vi "Create Grain.vi"(9 "Grain Size":T1={"Min Length (A)"=10.0, "Max Length (A)"=60.0, "Max Height"=100.0, "Max Width"=100.0, "Grain 1 Start"=0.0, "Tolerance"=0.1}, 10 "Viewing Angle":dbl[](array[numeric])=[1.0, -1.0, 0.0], 11 "Grain Orientation":dbl[](array[numeric])=[1.0, 1.0, 1.0]) -> (3 "Grain":T2={"Structure Name"="CdTe Expanded to Box", "Lattice vector a"=[10.01, 0.0, 0.0], "Lattice vector b"=[0.0, 10.01, 0.0], "Lattice vector c"=[0.0, 0.0, 11.3], "Atoms Array"=[{"Atom Name"="Cd", "Positions (Direct)"=[[0.0, 0.0, 0.0], [0.0, 0.26981849571539923, 0.67603992388645], [0.0, 0.5396369914307985, 0.338019961943225], [0.0, 0.8094554871461977, 0.0], [0.23366967170043837, 0.13490924785769962, 0.338019961943225], [0.23366967170043837, 0.4047277435730989, 0.0], [0.23366967170043837, 0.674546239288498, 0.67603992388645], [0.23366967170043837, 0.9443647350038973, 0.338019961943225], [0.46733934340087674, 0.0, 0.0], [0.46733934340087674, 0.26981849571539923, 0.67603992388645], [0.46733934340087674, 0.5396369914307986, 0.338019961943225], [0.46733934340087674, 0.8094554871461977, 0.0], [0.7010090151013151, 0.13490924785769962, 0.338019961943225], [0.7010090151013151, 0.4047277435730989, 0.0], [0.7010090151013151, 0.674546239288498, 0.67603992388645], [0.7010090151013151, 0.9443647350038973, 0.338019961943225], [0.9346786868017535, 0.0, 0.0], [0.9346786868017535, 0.26981849571539923, 0.67603992388645], [0.9346786868017535, 0.5396369914307985, 0.338019961943225], [0.9346786868017535, 0.8094554871461977, 0.0]], "Positions (Cartesian)"=[[0.0, 0.0, 0.0], [0.0, 2.700883142111146, 7.639251139916884], [0.0, 5.401766284222292, 3.819625569958442], [0.0, 8.10264942633344, 0.0], [2.339033413721388, 1.350441571055573, 3.819625569958442], [2.339033413721388, 4.05132471316672, 0.0], [2.339033413721388, 6.752207855277865, 7.639251139916884], [2.339033413721388, 9.453090997389012, 3.819625569958442], [4.678066827442776, 0.0, 0.0], [4.678066827442776, 2.700883142111146, 7.639251139916884], [4.678066827442776, 5.401766284222293, 3.819625569958442], [4.678066827442776, 8.10264942633344, 0.0], [7.017100241164163, 1.350441571055573, 3.819625569958442], [7.017100241164163, 4.05132471316672, 0.0], [7.017100241164163, 6.752207855277865, 7.639251139916884], [7.017100241164163, 9.453090997389012, 3.819625569958442], [9.356133654885552, 0.0, 0.0], [9.356133654885552, 2.700883142111146, 7.639251139916884], [9.356133654885552, 5.401766284222292, 3.819625569958442], [9.356133654885552, 8.10264942633344, 0.0]]}, {"Atom Name"="Te", "Positions (Direct)"=[[0.0, 0.0, 0.25351497145741875], [0.0, 0.2698184957153993, 0.9295548953438687], [0.0, 0.5396369914307985, 0.5915349334006437], [0.0, 0.8094554871461977, 0.25351497145741886], [0.23366967170043837, 0.1349092478576996, 0.5915349334006438], [0.23366967170043837, 0.40472774357309876, 0.25351497145741886], [0.23366967170043837, 0.674546239288498, 0.9295548953438687], [0.23366967170043837, 0.9443647350038973, 0.5915349334006438], [0.46733934340087674, 4.4364556428577685e-17, 0.25351497145741886], [0.46733934340087674, 0.26981849571539923, 0.9295548953438687], [0.46733934340087674, 0.5396369914307986, 0.5915349334006438], [0.46733934340087674, 0.8094554871461977, 0.25351497145741875], [0.7010090151013151, 0.1349092478576996, 0.5915349334006438], [0.7010090151013151, 0.40472774357309876, 0.25351497145741886], [0.7010090151013151, 0.674546239288498, 0.9295548953438687], [0.7010090151013151, 0.9443647350038973, 0.5915349334006438], [0.9346786868017535, 0.0, 0.25351497145741875], [0.9346786868017535, 0.2698184957153993, 0.9295548953438687], [0.9346786868017535, 0.5396369914307985, 0.5915349334006437], [0.9346786868017535, 0.8094554871461977, 0.25351497145741886]], "Positions (Cartesian)"=[[0.0, 0.0, 2.864719177468832], [0.0, 2.7008831421111466, 10.503970317385717], [0.0, 5.401766284222292, 6.684344747427274], [0.0, 8.10264942633344, 2.864719177468833], [2.339033413721388, 1.3504415710555728, 6.684344747427275], [2.339033413721388, 4.051324713166719, 2.864719177468833], [2.339033413721388, 6.752207855277865, 10.503970317385717], [2.339033413721388, 9.453090997389012, 6.684344747427275], [4.678066827442776, 4.440892098500626e-16, 2.864719177468833], [4.678066827442776, 2.700883142111146, 10.503970317385717], [4.678066827442776, 5.401766284222294, 6.684344747427275], [4.678066827442776, 8.10264942633344, 2.864719177468832], [7.017100241164163, 1.3504415710555728, 6.684344747427275], [7.017100241164163, 4.051324713166719, 2.864719177468833], [7.017100241164163, 6.752207855277865, 10.503970317385717], [7.017100241164163, 9.453090997389012, 6.684344747427275], [9.356133654885552, 0.0, 2.864719177468832], [9.356133654885552, 2.7008831421111466, 10.503970317385717], [9.356133654885552, 5.401766284222292, 6.684344747427274], [9.356133654885552, 8.10264942633344, 2.864719177468833]]}], "# of atoms"=40} {"Atoms Array"."Positions (Cartesian)" format="%#_4f"; "Atoms Array"."Positions (Direct)" format="%#_4f"})   [LabVIEW 2010]
uses:
  <vilib>/Analysis/_algsub.llb/Real Vector Norm.vi
  <vilib>/Analysis/NI_AALPro.lvlib
panel:
  in  "Conventional Unit Cell":T2={"Structure Name"="CdTe", "Lattice vector a"=[6.615785553057252, 0.0, 0.0], "Lattice vector b"=[0.0, 6.615785553057252, 0.0], "Lattice vector c"=[0.0, 0.0, 6.615785553057252], "Atoms Array"=[{"Atom Name"="Cd", "Positions (Direct)"=[[0.0, 0.0, 0.0], [0.0, 0.5, 0.5], [0.5, 0.0, 0.5], [0.5, 0.5, 0.0]], "Positions (Cartesian)"=[[0.0, 0.0, 0.0], [0.0, 3.307892776528626, 3.307892776528626], [3.307892776528626, 0.0, 3.307892776528626], [3.307892776528626, 3.307892776528626, 0.0]]}, {"Atom Name"="Te", "Positions (Direct)"=[[0.25, 0.25, 0.25], [0.75, 0.75, 0.25], [0.75, 0.25, 0.75], [0.25, 0.75, 0.75]], "Positions (Cartesian)"=[[1.653946388264313, 1.653946388264313, 1.653946388264313], [4.96183916479294, 4.96183916479294, 1.653946388264313], [4.96183916479294, 1.653946388264313, 4.96183916479294], [1.653946388264313, 4.96183916479294, 4.96183916479294]]}], "# of atoms"=8}
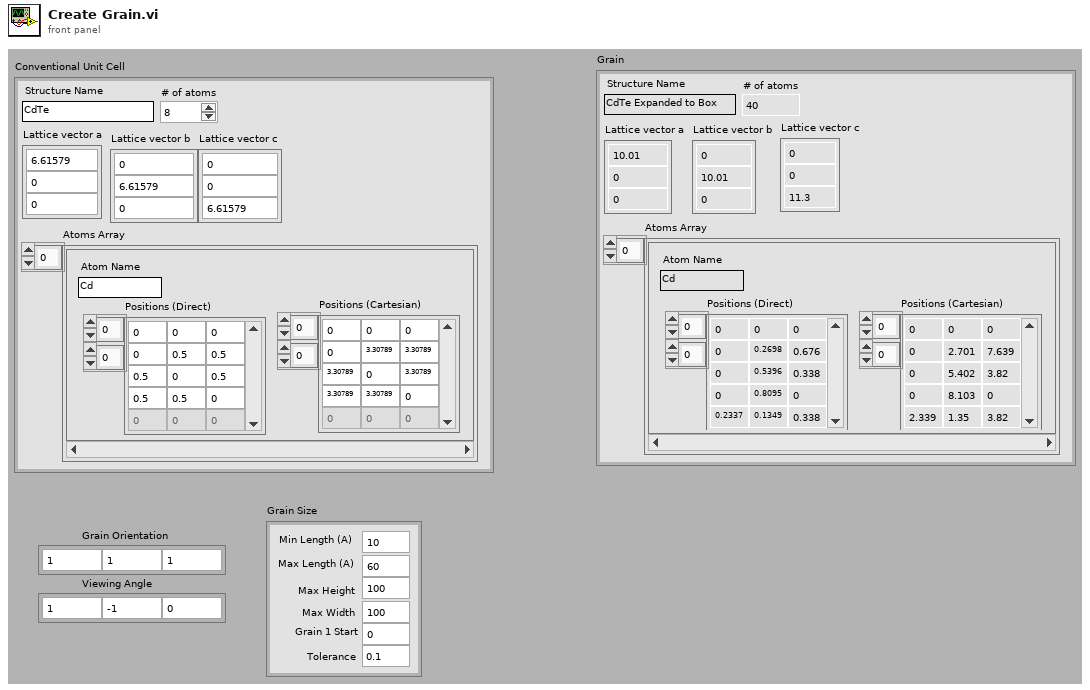
[diagram p1: front panel]
types:
  T1 = cluster{"Min Length (A)":dbl, "Max Length (A)":dbl, "Max Height":dbl, "Max Width":dbl, "Grain 1 Start":dbl, "Tolerance":dbl}
  T2 = cluster{"Structure Name":string, "Lattice vector a":dbl[], "Lattice vector b":dbl[], "Lattice vector c":dbl[], "Atoms Array":cluster{"Atom Name":string, "Positions (Direct)":dbl[][], "Positions (Cartesian)":dbl[][]}[], "# of atoms":i32}
  T3 = typedef "NI_Matrix.lvlib/RealMatrix.ctl" = dbl[][]
  T4 = cluster{dbl, "Max Width":dbl, dbl, "Max Height":dbl, "Grain 1 Start":dbl, "Max Length (A)":dbl}
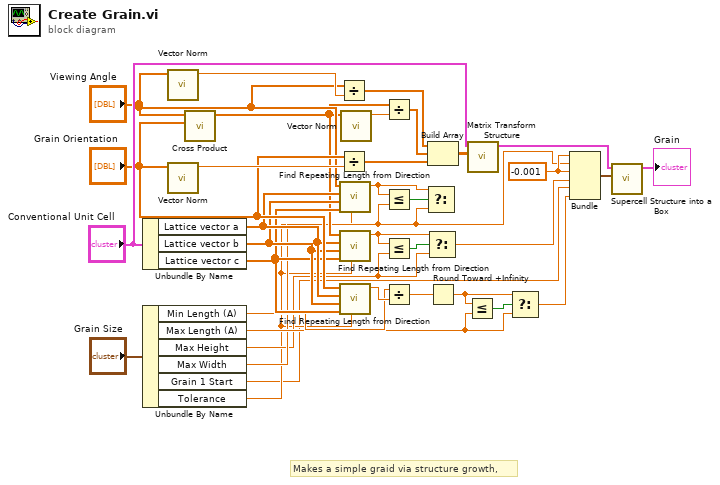
[diagram p0: block diagram]
diagram:
  w10 = -0.001
  # "Makes a simple graid via structure growth,"
  n1 = Unbundle By Name("Conventional Unit Cell") -> ("Lattice vector a"=w21:dbl[], "Lattice vector b"=w20:dbl[], "Lattice vector c"=w19:dbl[])
  n2 = Unbundle By Name("Grain Size") -> ("Min Length (A)"=w6:dbl, "Max Length (A)"=w5:dbl, "Max Height"=w3:dbl, "Max Width"=w4:dbl, "Grain 1 Start"=w1:dbl, "Tolerance"=w2:dbl)
  n3 = call-poly <vilib>:"Vector Norm.vi"("Input Vector"="Viewing Angle") -> ("norm"=w35:dbl)  [unwired: 9 in, 1 out]
  n4 = call-poly <vilib>:"Vector Norm.vi"("Input Vector"="Grain Orientation") -> ("norm"=w33:dbl)  [unwired: 9 in, 1 out]
  n5 = call <vilib>:"Cross Product.vi"("B Vector"="Grain Orientation", "A Vector"="Viewing Angle") -> ("Cross Product"=w17:dbl[])  [unwired: 8 in, 1 out]
  n6 = Divide(x="Viewing Angle", y=w35) -> (x/y=w32:dbl[])
  n7 = Divide(x="Grain Orientation", y=w33) -> (x/y=w31:dbl[])
  n8 = call "Find Repeating Length from Direction.vi"("Tolerance"=w2, "Lattice vector c"=w19, "Lattice vector b"=w20, "Lattice vector a"=w21, "Direction"="Viewing Angle") -> ("Repeating Length (A)"=w15:dbl)  [unwired: 6 in]
  n9 = call "Find Repeating Length from Direction.vi"("Tolerance"=w2, "Lattice vector c"=w19, "Lattice vector b"=w20, "Lattice vector a"=w21, "Direction"=w17) -> ("Repeating Length (A)"=w13:dbl)  [unwired: 6 in]
  n10 = call "Find Repeating Length from Direction.vi"("Tolerance"=w2, "Lattice vector c"=w19, "Lattice vector b"=w20, "Lattice vector a"=w21, "Direction"="Grain Orientation") -> ("Repeating Length (A)"=w25:dbl)  [unwired: 6 in]
  n11 = call-poly <vilib>:"Vector Norm.vi"("Input Vector"=w17) -> ("norm"=w34:dbl)  [unwired: 9 in, 1 out]
  n12 = Divide(x=w17, y=w34) -> (x/y=w28:dbl[])
  n13 = Less Or Equal?(x=w15, y=w4) -> (x <= y?=w16:bool)
  n14 = Less Or Equal?(x=w13, y=w3) -> (x <= y?=w14:bool)
  n15 = Divide(x=w6, y=w25) -> (x/y=w24:dbl)
  n16 = Select(t=w15, s=w16, f=w4) -> ()  [unwired: 1 out]
  n17 = Select(t=w13, s=w14, f=w3) -> (s? t:f=w12:dbl)
  n18 = Build Array(w32, w28, w31) -> (w30:T3)
  n19 = Round Toward +Infinity(x=w24) -> (ceil(x): smallest int >= x=w22:dbl)
  n20 = Less Or Equal?(x=w22, y=w5) -> (x <= y?=w23:bool)
  n21 = call "Matrix Transform Structure.vi"("Matrix Transform"=w30, "Original Structure"="Conventional Unit Cell") -> ("After Transform"=w29:T2)  [unwired: 9 in]
  n22 = Select(t=w22, s=w23, f=w5) -> (s? t:f=w11:dbl)
  n23 = Bundle(w10, "Max Width"=w4, w10, "Max Height"=w12, "Grain 1 Start"=w1, "Max Length (A)"=w11) -> (w9:T4)  [unwired: 1 in]
  n24 = call "Supercell Structure into a Box.vi"("Draw Box"=w9, "Subcrystal"=w29) -> ("Expanded cubic Structure"=→"Grain":T2)  [unwired: 7 in, 2 out]
